vi "Sort 2D string Array.vi"(8 "error in (no error)":errorcluster, 9 "Descending (F)":bool, 10 "Priority Columns (0)":i32[](array[numeric])=[0], 11 "Unsorted Array":string[][](array[string])) -> (0 "error out":errorcluster, 2 "Sorted array using numbers":string[][](array[string]), 3 "Sorted array":string[][](array[string]))   [LabVIEW 2013]
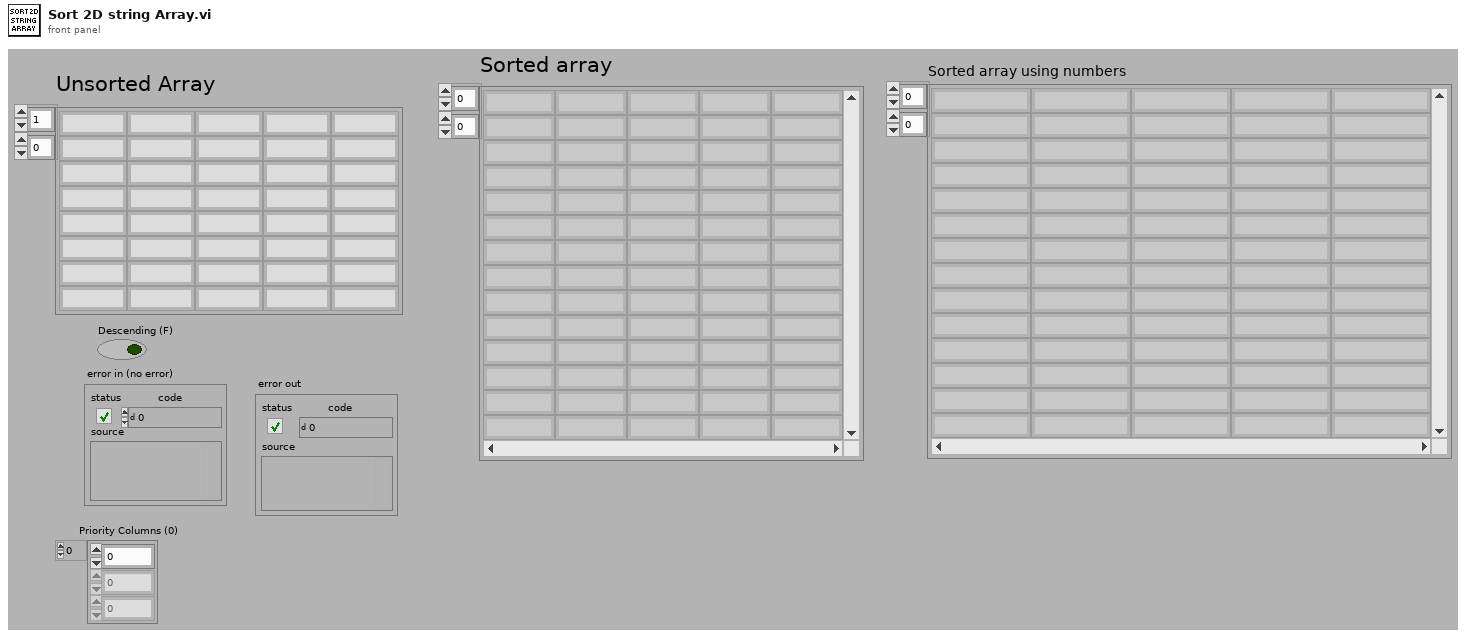
[diagram p1: front panel]
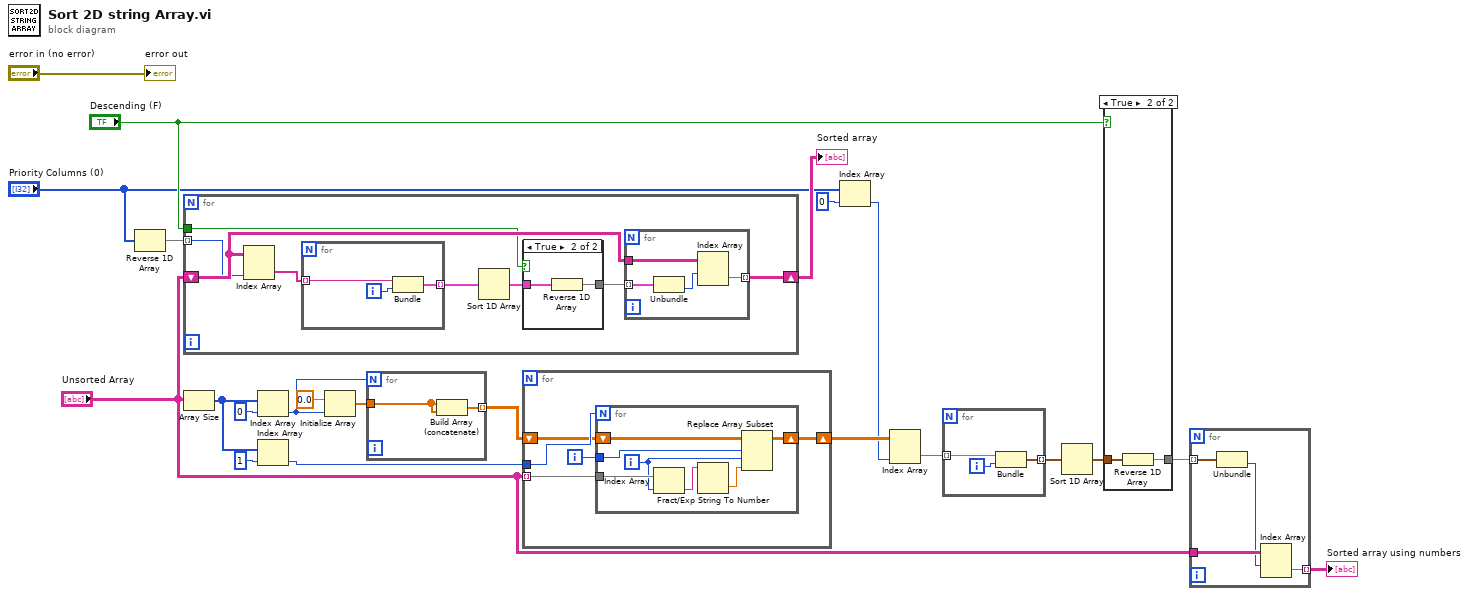
[diagram p0: block diagram]
diagram:
  n1 = Reverse 1D Array(array="Priority Columns (0)") -> (reversed array=w22:i32[])
  n2 = for {
    shift-right: [w24] -> w21
    shift-left: "Unsorted Array" -> [w26]
    tunnel: w22 -> [w23] mode=indexing
    tunnel: "Descending (F)" -> [w25]
    n3 = Index Array(array=w26, index (col)=w23) -> (element=w28:string[])  [unwired: 1 in]
    n4 = for {
      tunnel: w28 -> [w38] mode=indexing
      tunnel: [w40] -> w27 mode=indexing
      i -> [w39]
      n5 = Bundle("String"=w38, w39) -> (w40:cluster{"String":string, i32})  [unwired: 1 out]
    }
    n6 = Sort 1D Array(array=w27) -> (sorted array=w30:cluster{"String":string, i32}[])
    n7 = case shown="True" w25 {
      tunnel: [w31 w32] -> w29
      tunnel: w30 -> [w31 w33]
      frame False {
      }
      frame True {
        n8 = Reverse 1D Array(array=w33) -> (reversed array=w32:cluster{"String":string, i32}[])
      }
    }
    n9 = for {
      tunnel: w29 -> [w37] mode=indexing
      tunnel: w26 -> [w36]
      tunnel: [w34] -> w24 mode=indexing
      n10 = Unbundle(w37) -> (w35:i32)  [unwired: 1 out]
      n11 = Index Array(array=w36, index (row)=w35) -> (element=w34:string[])  [unwired: 1 in]
    }
  }
  "Sorted array" <- w21
  n12 = Array Size(array="Unsorted Array") -> (size(s)=w16:i32[])
  n13 = Index Array(array=w16, index=0) -> (element=w14:i32)
  n14 = Index Array(array=w16, index=1) -> (element=w18:i32)
  n15 = Initialize Array(0.0, w14) -> (w13:dbl[])
  n16 = for {
    N: w14 -> [_]
    tunnel: w13 -> [w42]
    tunnel: [w41] -> w12 mode=indexing
    n17 = Build Array (concatenate)(w42, w42) -> (w41:dbl[])
  }
  n18 = for {
    tunnel: "Unsorted Array" -> [w46] mode=indexing
    tunnel: w18 -> [w47]
    shift-right: [w43] -> w8
    shift-left: w12 -> [w45]
    i -> [w44]
    n19 = for {
      N: w47 -> [_]
      tunnel: w46 -> [w54]
      tunnel: w44 -> [w51]
      shift-right: [w50] -> w43
      shift-left: w45 -> [w52]
      i -> [w48]
      n20 = Index Array(array=w54, index=w48) -> (element=w53:string)
      n21 = Fract/Exp String To Number(string=w53) -> (number=w49:dbl)  [unwired: 3 in, 1 out]
      n22 = Replace Array Subset(array=w52, new element=w49, index (row)=w51, index (col)=w48) -> (w50:dbl[][])
    }
  }
  n23 = Index Array(array="Priority Columns (0)", index=0) -> (element=w1:i32)
  n24 = Index Array(array=w8, index (col)=w1) -> (element=w10:dbl[])  [unwired: 1 in]
  n25 = for {
    tunnel: w10 -> [w55] mode=indexing
    tunnel: [w57] -> w9 mode=indexing
    i -> [w56]
    n26 = Bundle(w55, w56) -> (w57:cluster{dbl, i32})  [unwired: 1 out]
  }
  n27 = Sort 1D Array(array=w9) -> (sorted array=w11:cluster{dbl, i32}[])
  n28 = case shown="True" "Descending (F)" {
    tunnel: [w58 w59] -> w5
    tunnel: w11 -> [w58 w60]
    frame False {
    }
    frame True {
      n29 = Reverse 1D Array(array=w60) -> (reversed array=w59:cluster{dbl, i32}[])
    }
  }
  n30 = for {
    tunnel: w5 -> [w64] mode=indexing
    tunnel: "Unsorted Array" -> [w63]
    tunnel: [w61] -> w4 mode=indexing
    n31 = Unbundle(w64) -> (w62:i32)  [unwired: 1 out]
    n32 = Index Array(array=w63, index (row)=w62) -> (element=w61:string[])  [unwired: 1 in]
  }
  "Sorted array using numbers" <- w4
  "error out" <- "error in (no error)"
